vi "FW_parse_Results_data.vi"(7 "?":T6={"Py session"=refnum, "BirdEyeView_params"={"P1"={"x"=970, "y"=485}, "P2"={"x"=0, "y"=750}, "Alfa"=6.0}, "frames_Result"=[]}, 8 "Warpped_detected_points":cluster{"X":sgl, "Y":sgl}[][](array[cluster]), 9 "Image_Warpped_BW":T3, 10 "Image_Warp_perspective":T3, 11 "Payload_cluster":T5) -> (3 "consumer_loop":T6={"Py session"=refnum, "BirdEyeView_params"={"P1"={"x"=970, "y"=485}, "P2"={"x"=0, "y"=750}, "Alfa"=6.0}, "frames_Result"=[]})   [LabVIEW 2021, in "Framework_lib.lvlib"]
uses:
  QMH/Framework_lib.lvlib
  FW_Results_Data.ctl
  FW_Frames_Data.ctl
  QMH/QMH_Producer_type.ctl
  FW_Image_resultant_data.ctl
  <vilib>/vision/Image Controls.llb/IMAQ Image.ctl
  QMH/QMH_references_enum.ctl
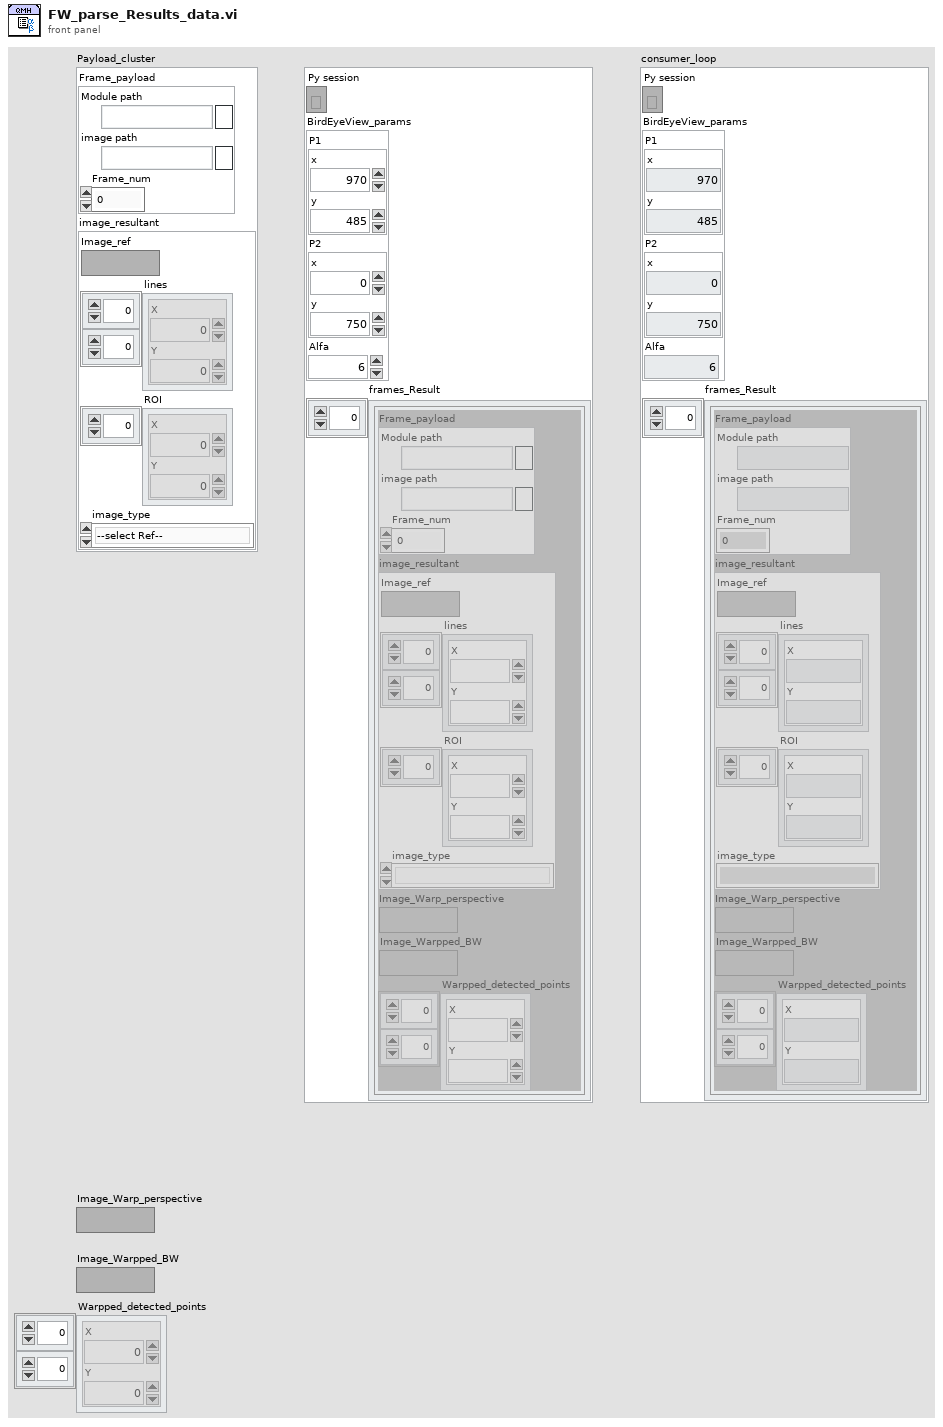
[diagram p1: front panel]
types:
  T1 = typedef "Framework_lib.lvlib/QMH_Producer_type.ctl" = cluster{"Module path":path, "image path":path, "Frame_num":u16}
  T2 = typedef "Framework_lib.lvlib/FW_Image_resultant_data.ctl" = cluster{"Image_ref":T3, "lines":cluster{"X":dbl, "Y":dbl}[][], "ROI":cluster{"X":dbl, "Y":dbl}[], "image_type":T4}
  T3 = typedef "IMAQ Image.ctl" = refnum<image>
  T4 = typedef "Framework_lib.lvlib/QMH_references_enum.ctl" = enum16{"--select Ref--", "Consumer_SUT", "Consumer_Annot", "Compute_Results"}
  T5 = cluster{"Frame_payload":T1, "image_resultant":T2}
  T6 = typedef "Framework_lib.lvlib/FW_Results_Data.ctl" = cluster{"Py session":refnum<k35>, "BirdEyeView_params":cluster{"P1":cluster{"x":i16, "y":i16}, "P2":cluster{"x":i16, "y":i16}, "Alfa":dbl}, "frames_Result":T7[]}
  T7 = typedef "Framework_lib.lvlib/FW_Frames_Data.ctl" = cluster{"Frame_payload":T1, "image_resultant":T2, "Image_Warp_perspective":T3, "Image_Warpped_BW":T3, "Warpped_detected_points":cluster{"X":sgl, "Y":sgl}[][]}
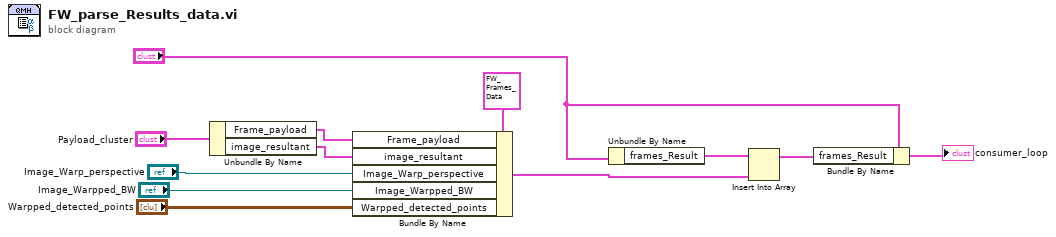
[diagram p0: block diagram]
diagram:
  n1 = Unbundle By Name("Payload_cluster") -> ("Frame_payload"=w4:T1, "image_resultant"=w3:T2)
  n2 = Bundle By Name(cluster=T7 {"Frame_payload"={"Module path"=path "", "image path"=path "", "Frame_num"=0}, "image_resultant"={"Image_ref"=refnum, "lines"=[], "ROI"=[], "image_type"=enum."--select Ref--"}, "Image_Warp_perspective"=refnum, "Image_Warpped_BW"=refnum, "Warpped_detected_points"=[[{"X"=0.0, "Y"=0.0}, {"X"=0.0, "Y"=0.0}], [{"X"=0.0, "Y"=0.0}, {"X"=0.0, "Y"=0.0}]]} ("Cluster"), "Frame_payload"=w4, "image_resultant"=w3, "Image_Warp_perspective"="Image_Warp_perspective", "Image_Warpped_BW"="Image_Warpped_BW", "Warpped_detected_points"="Warpped_detected_points") -> (w8:T7)
  n3 = Unbundle By Name("?") -> ("frames_Result"=w2:T7[])
  n4 = Insert Into Array(array=w2, new element=w8) -> (w1:T7[])  [unwired: 1 in]
  n5 = Bundle By Name(cluster="?", "frames_Result"=w1) -> (→"consumer_loop":T6)
